vi "Test TDMS.vi"() -> ()   [LabVIEW 2014]
panel:
  in  "Multicolumn Listbox":i32(listbox)
  in  "Channel Names":i32(listbox)
  in  "Group Names":i32(listbox)
  out "Number of data":i64
  in  "stop 2":bool
  out "waveform out":waveform(dbl)
  in  "Slide":dbl(slide) scale=0.0..1.0
  in  "file path":path
  in  "stop":bool
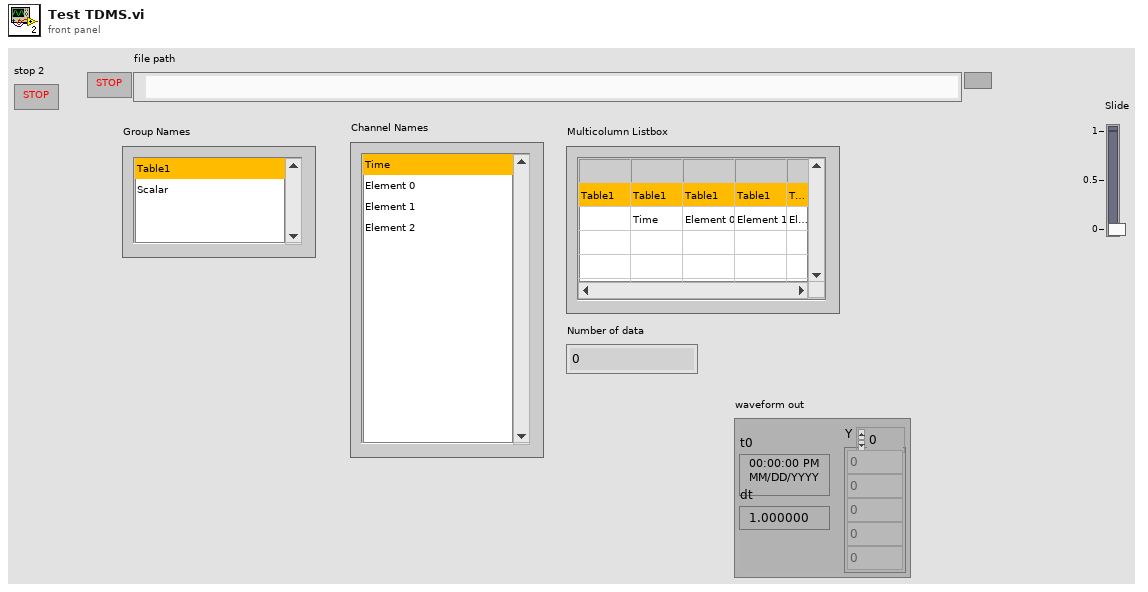
[diagram p1: front panel]
types:
  T1 = enum16{"open", "open or create", "create or replace", "create", "open (read-only)"}
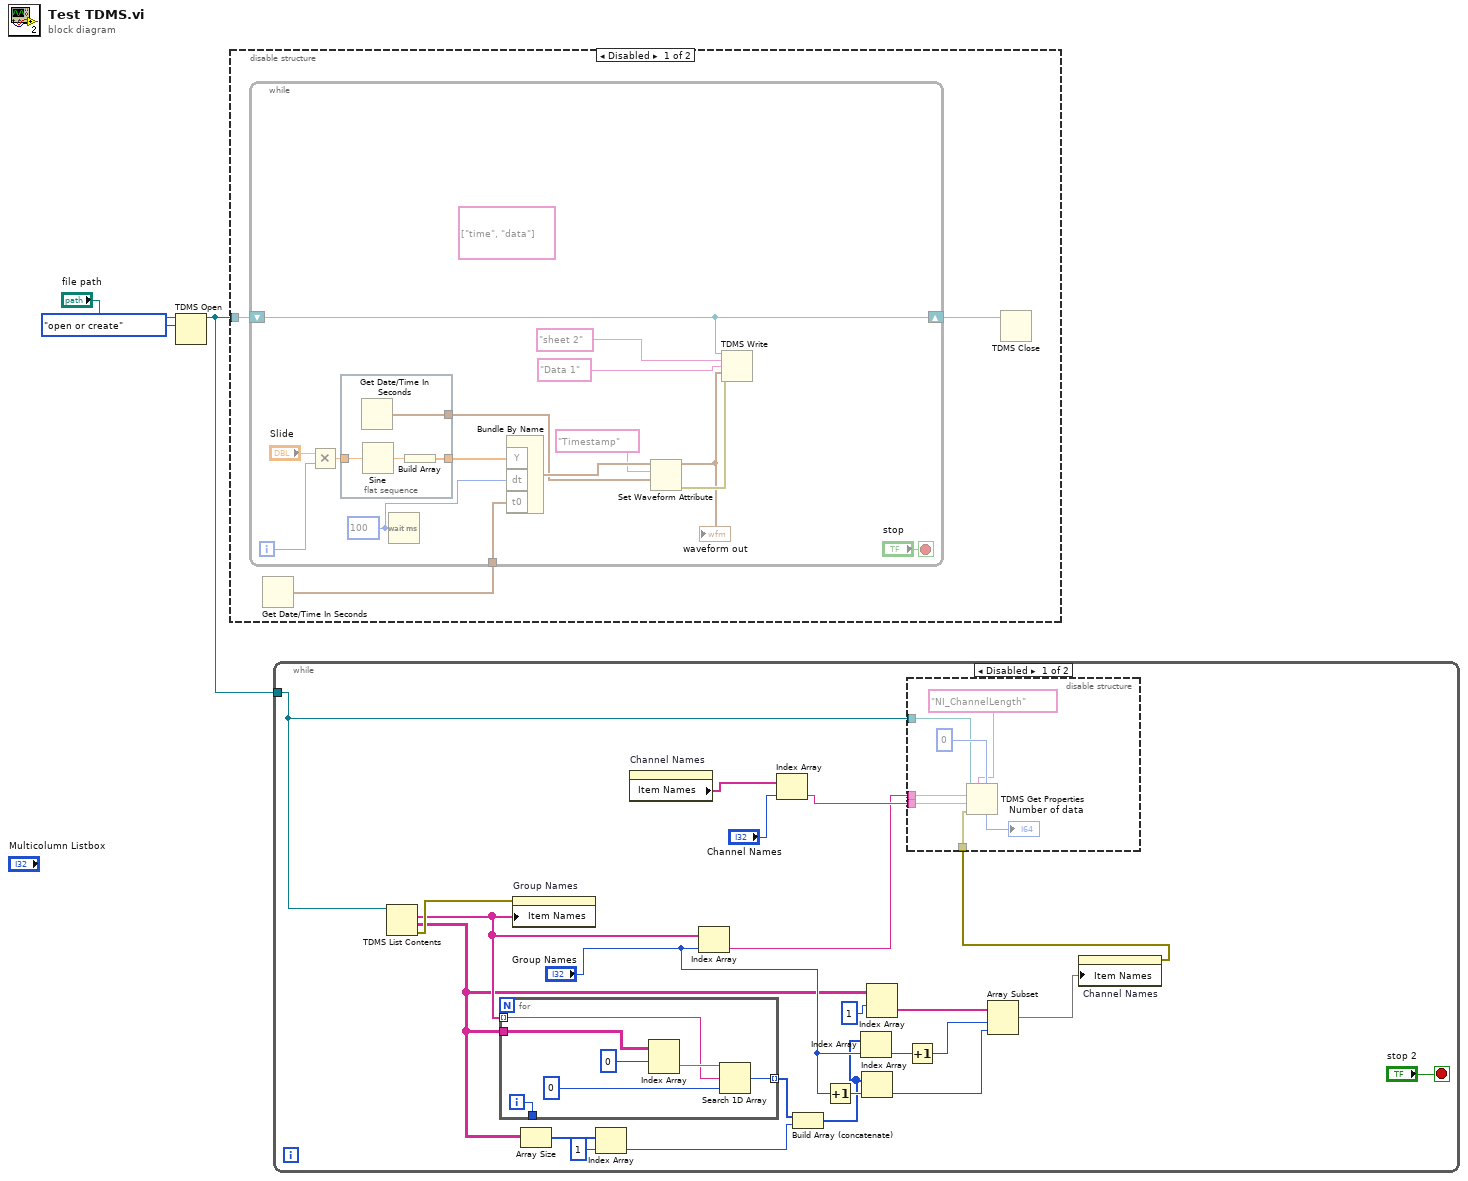
[diagram p0: block diagram]
diagram:
  n1 = TDMS Open(10:T1."open or create" ("operation (0:open)"), 11:"file path") -> (3:w1:refnum<k34>)  [unwired: 5 in, 1 out]
  n2 = disable-structure shown="Disabled" {
    disable-tunnel: w1 -> [w4 _]
    frame Disabled {
      n3 = Get Date/Time In Seconds() -> (seconds since 1Jan1904=w5:timestamp)
      n4 = while {
        shift-right: [w14] -> w6
        shift-left: w4 -> [w14]
        tunnel: w5 -> [w12]
        i -> [w20]
        stop <- "stop" stop-if-true
        (unwired) string[] ["time", "data"]
        w17 = u32 100 ("milliseconds to wait")
        n5 = Multiply(x="Slide", y=w20) -> (x*y=w19:dbl)
        n6 = flat-sequence {
          tunnel: w19 -> [w25]
          tunnel: [w23] -> w7
          tunnel: [w22] -> w10
          frame #0 {
            n7 = Get Date/Time In Seconds() -> (seconds since 1Jan1904=w22:timestamp)
            n8 = Sine(x=w25) -> (sin(x)=w24:dbl)
            n9 = Build Array(w24) -> (w23:dbl[])
          }
        }
        n10 = Wait (ms)(milliseconds to wait=w17) -> ()  [unwired: 1 out]
        n11 = Bundle By Name("Y"=w7, "dt"=w17, "t0"=w12) -> (w16:waveform(dbl))  [unwired: 1 in]
        n12 = Set Waveform Attribute(5:w10, 6:"Timestamp" ("name"), 7:w16) -> (0:w13:errorcluster, 3:w8:waveform(dbl))  [unwired: 1 in, 1 out]
        "waveform out" <- w8
        n13 = TDMS Write(0:w14, 5:"sheet 2" ("name"), 7:"Data 1" ("name"), 9:w8, 11:w13) -> ()  [unwired: 1 in, 4 out]
      }
      n14 = TDMS Close(11:w6) -> ()  [unwired: 1 in, 2 out]
    }
    frame Enabled {
    }
  }
  n15 = while {
    tunnel: w1 -> [w47]
    stop <- "stop 2" stop-if-true
    n16 = TDMS List Contents(7:w47) -> (0:w46:errorcluster, 1:w34:string[][], 2:w45:string[])  [unwired: 2 in, 1 out]
    n17 = for {
      tunnel: w34 -> [w62]
      tunnel: w45 -> [w58] mode=indexing
      tunnel: [w57] -> w37 mode=indexing
      tunnel: [w56] -> _
      i -> [w56]
      n18 = Index Array(array=w62, index (row)=0) -> (element=w59:string[])  [unwired: 1 in]
      n19 = Search 1D Array(1D array=w59, element=w58, start index (0)=0 ("index (row)")) -> (index of element=w57:i32)
    }
    n20 = property on="Group Names" class="LstBox (strict)"(error in=w46, "Item Names"=w45) -> ()  [unwired: 1 in, 2 out]
    n21 = Array Size(array=w34) -> (size(s)=w33:i32[])
    n22 = Index Array(array=w33, index=1) -> (element=w31:i32)
    n23 = property on="Channel Names" class="LstBox (strict)"() -> ("Item Names"=w29:string[])  [unwired: 2 in, 2 out]
    n24 = Index Array(array=w45, index="Group Names") -> (element=w26:string)
    n25 = Index Array(array=w29, index="Channel Names") -> (element=w27:string)
    n26 = Build Array (concatenate)(w37, w31) -> (w36:i32[])
    n27 = Increment(x="Group Names") -> (x+1=w40:i32)
    n28 = Index Array(array=w36, index="Group Names") -> (element=w42:i32)
    n29 = Index Array(array=w36, index=w40) -> (element=w38:i32)
    n30 = Index Array(array=w34, index (row)=1 ("disabled index (col)")) -> (element=w44:string[])  [unwired: 1 in]
    n31 = Increment(x=w42) -> (x+1=w41:i32)
    n32 = Array Subset(array=w44, index=w41, length=w38) -> (w35:string[])
    n33 = property on="Channel Names" class="LstBox (strict)"("Item Names"=w35) -> (error out=w30:errorcluster)  [unwired: 2 in, 1 out]
    n34 = disable-structure shown="Disabled" {
      disable-tunnel: w47 -> [w53 _]
      disable-tunnel: w30 -> [w51 _]
      disable-tunnel: w27 -> [w50 _]
      disable-tunnel: w26 -> [w49 _]
      frame Disabled {
        n35 = TDMS Get Properties(5:i64 0, 7:"NI_ChannelLength" ("channel name(s) in"), 8:w51, 9:w50, 10:w49, 11:w53) -> (4:→"Number of data":i64)  [unwired: 5 out]
      }
      frame Enabled {
      }
    }
  }
